vi "Get_Next_Sub_Collection.vi"(8 "error in (no error)":errorcluster caption="entrée d'erreur (pas d'erreur)", 11 "Firebase Benches en entrée":refnum<class "Firebase Benches.lvclass">) -> (0 "error out":errorcluster caption="sortie d'erreur", 3 "Firebase Benches en sortie":refnum<class "Firebase Benches.lvclass">)   [LabVIEW 2020, in "Library Instrument & Equipement.lvlib" / "Library FireBase.lvlib" / "Firebase Benches.lvclass"]
doc: "Return the documents present in the test collection for each DATA read with Get_Data\nPlease initialise the following values\n - Name BDD\n - Document of test sequence\n - API Key\n - Nb To Read"
uses:
  Firebase Benches.lvclass
  C:/Users/ngarcin/OneDrive - Altyor/Standard TB/Class/Firebase/Source/Firebase Driver/Firebase Driver.lvclass
  Firebase Altyor/Firebase Altyor.lvclass
  Firebase Benches.lvclass/Firebase Benches.ctl
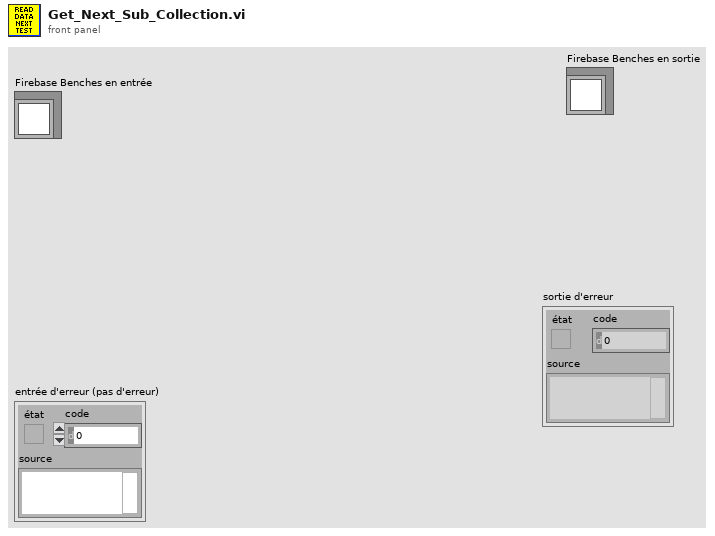
[diagram p1: front panel]
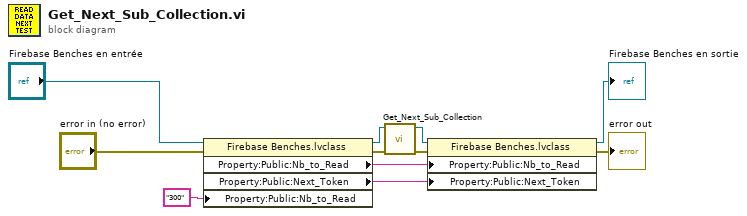
[diagram p0: block diagram]
diagram:
  n1 = property class="Firebase Benches.lvclass"(reference="Firebase Benches en entrée", error in="error in (no error)", "Property:Public:Nb_to_Read"="300" ("Nb_to_Read")) -> (reference out=w5:refnum<class "Firebase Benches.lvclass">, error out=w8:errorcluster, "Property:Public:Nb_to_Read"=w11:string, "Property:Public:Next_Token"=w9:string)
  n2 = call-parent "Get_Next_Sub_Collection.vi"("error in (no error)"=w8, "Firebase Altyor en entrée"=w5) -> ("error out"=w7:errorcluster, "Firebase Altyor en sortie"=w6:refnum<class "Firebase Benches.lvclass">)  [unwired: 8 in]
  n3 = property class="Firebase Benches.lvclass"(reference=w6, error in=w7, "Property:Public:Nb_to_Read"=w11, "Property:Public:Next_Token"=w9) -> (reference out=→"Firebase Benches en sortie":refnum<class "Firebase Benches.lvclass">, error out=→"error out":errorcluster)
